vi "replace shot number in tcp reply.vi"(10 ">>new shot#string>>":string=">>NaN>>", 11 "input string":string) -> (3 "result string":string)   [LabVIEW 2020]
uses:
  Match Regular Expression.xnode
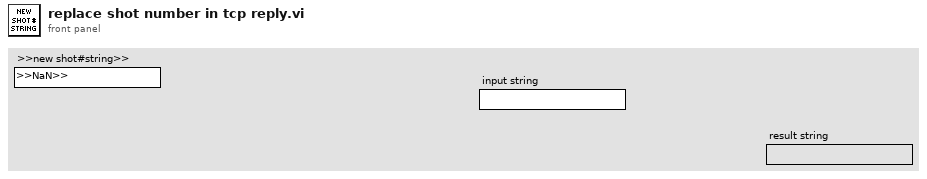
[diagram p1: front panel]
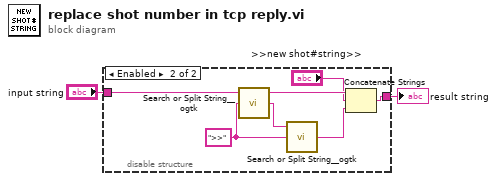
[diagram p0: block diagram]
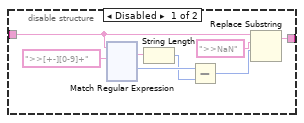
[diagram p2: hidden frame]
diagram:
  n1 = disable-structure shown="Enabled" {
    disable-tunnel: "input string" -> [w9 w131]
    disable-tunnel: [w7 w125] -> w1
    frame Disabled {
      n2 = xnode "Match Regular Expression"("input string"=w9, "regular expression"=">>[+-][0-9]+") -> ("whole match"=w6:string, "offset past match"=w5:i32)  [unwired: 4 in, 3 out]
      n3 = String Length(string=w6) -> (length=w4:i32)
      n4 = Subtract(x=w5, y=w4) -> (x-y=w3:i32)
      n5 = Replace Substring(3:w3, 4:">>NaN" ("substring (\"\")"), 5:w9) -> (1:w7:string)  [unwired: 1 in, 1 out]
    }
    frame Enabled {
      w129 = ">>" ("search string/char (-)")
      n6 = call "Search or Split String__ogtk.vi"("search string/char (-)"=w129, "string"=w131) -> ("substring after match"=w130:string, "substring before match"=w128:string)  [unwired: 1 in, 1 out]
      n7 = call "Search or Split String__ogtk.vi"("search string/char (-)"=w129, "string"=w130) -> ("substring after match"=w126:string)  [unwired: 1 in, 2 out]
      n8 = Concatenate Strings(w128, ">>new shot#string>>", w126) -> (w125:string)
    }
  }
  "result string" <- w1
